vi "mxwScript_API_Option_GenericCleanupOption.vi"(7 "cleanupOption":string, 8 "error in (no error)":errorcluster, 9 "data":string, 10 "time":i32, 11 "options in":T1[](array[typedef])) -> (0 "error out":errorcluster, 3 "options out":T1[](array[typedef]))   [LabVIEW 2017]
uses:
  codeGenAPISupport.llb/cgAPI_mxwScript_OptionData.ctl
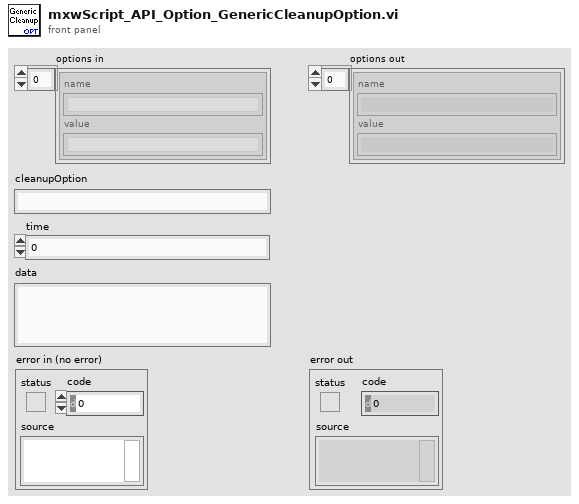
[diagram p1: front panel]
types:
  T1 = typedef "cgAPI_mxwScript_OptionData.ctl" = cluster{"name":string, "value":string}
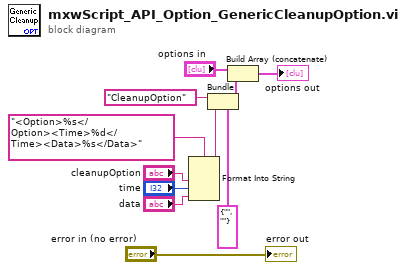
[diagram p0: block diagram]
diagram:
  n1 = Format Into String(format string="<Option>%s</Option><Time>%d</Time><Data>%s</Data>", "cleanupOption", "time", "data") -> (resulting string=w6:string)  [unwired: 2 in, 1 out]
  n2 = Bundle(cluster=T1 {"name"="", "value"=""} ("optionData"), "name"="CleanupOption", "value"=w6) -> (w10:T1)
  n3 = Build Array (concatenate)("options in", w10) -> (→"options out":T1[])
  "error out" <- "error in (no error)"
